vi "Receive Results Object.vi"(8 "error in (no error)":errorcluster, 10 "Results.lvclass":refnum<class "Results.lvclass">, 11 "Controller in":refnum<class "Controller.lvclass">) -> (0 "error out":errorcluster, 3 "Controller out":refnum<class "Controller.lvclass">)   [LabVIEW 2015, in "Controller Actor.lvlib" / "Controller.lvclass"]
uses:
  Controller.lvclass
  Results/Results.lvclass
  Results/Results.lvclass/Results.ctl
  <vilib>/ActorFramework/Message Enqueuer/Message Enqueuer.lvclass/Message Enqueuer.ctl
  <vilib>/ActorFramework/Message Enqueuer/Enqueue.vi
  <vilib>/ActorFramework/Message Priority Queue/Priority Enqueue.vi
  <vilib>/ActorFramework/Stop Msg/Stop Msg.lvclass
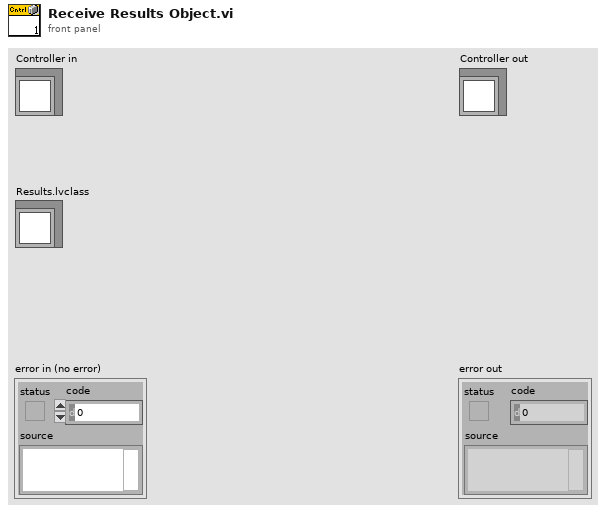
[diagram p1: front panel]
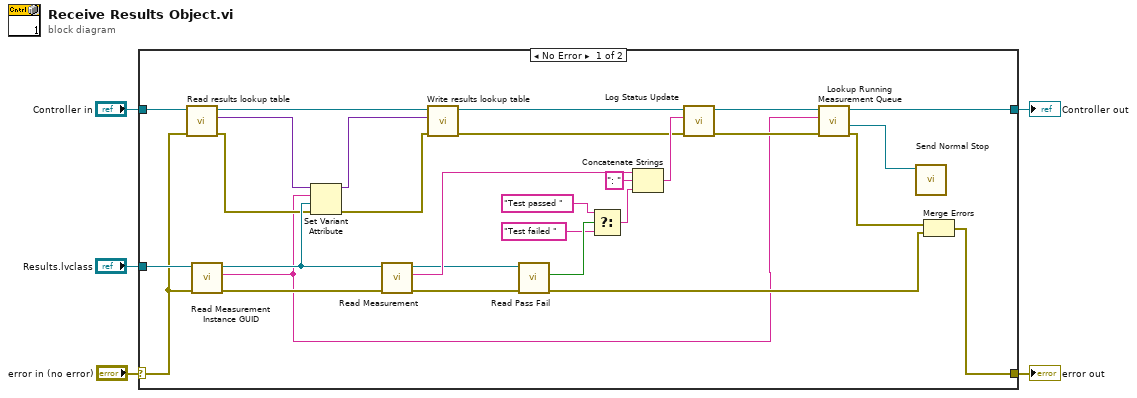
[diagram p0: block diagram]
diagram:
  n1 = case shown="No Error" "error in (no error)" {
    selector: "error in (no error)" -> [w6 w36]
    tunnel: [w9 w36] -> w4
    tunnel: [w19 w35] -> w2
    tunnel: "Controller in" -> [w8 w35]
    tunnel: "Results.lvclass" -> [w21 _]
    frame No Error {
      n2 = call "Read results lookup table.vi"("error in (no error)"=w6, "Controller in"=w8) -> ("error out"=w17:errorcluster, "results lookup table (measurement.timestamp -> results object)"=w34:variant, "Controller out"=w33:refnum<class "Controller.lvclass">)  [unwired: 7 in]
      n3 = call "Read Measurement Instance GUID.vi"("error in (no error)"=w6, "Results in"=w21) -> ("error out"=w13:errorcluster, "Measurement Instance GUID"=w7:string, "Results out"=w31:refnum<class "Results.lvclass">)  [unwired: 7 in]
      n4 = Set Variant Attribute(Variant=w34, name=w7, value=w31, error in=w17) -> (Variant out=w32:variant, error out=w16:errorcluster)  [unwired: 1 out]
      n5 = call "Read Measurement.vi"("error in (no error)"=w13, "Results in"=w31) -> ("error out"=w12:errorcluster, "Measurement"=w28:string, "Results out"=w27:refnum<class "Results.lvclass">)  [unwired: 7 in]
      n6 = call "Write results lookup table.vi"("error in (no error)"=w16, "results lookup table (measurement.timestamp -> results object)"=w32, "Controller in"=w33) -> ("error out"=w15:errorcluster, "Controller out"=w30:refnum<class "Controller.lvclass">)  [unwired: 7 in]
      n7 = call "Read Pass Fail.vi"("error in (no error)"=w12, "Results in"=w27) -> ("error out"=w11:errorcluster, "Pass Fail"=w24:bool)  [unwired: 7 in, 1 out]
      n8 = Select(t="Test passed " ("string"), s=w24, f="Test failed " ("string")) -> (s? t:f=w25:string)
      n9 = Concatenate Strings(w28, ": " ("string"), w25) -> (w29:string)
      n10 = call-dynamic "Log Status Update.vi"("error in (no error)"=w15, "String"=w29, "Controller in"=w30) -> ("error out"=w14:errorcluster, "Controller out"=w20:refnum<class "Controller.lvclass">)  [unwired: 7 in]
      n11 = call "Lookup Running Measurement Queue.vi"("error in (no error)"=w14, "Measurement Name.Harware()"=w7, "Controller in"=w20) -> ("error out"=w10:errorcluster, "Measurement Queue"=w18:refnum<class "Message Enqueuer.lvclass">, "Controller out"=w19:refnum<class "Controller.lvclass">)  [unwired: 5 in, 1 out]
      n12 = call <vilib>:"Send Normal Stop.vi"("Message Enqueuer"=w18) -> ()  [unwired: 10 in, 1 out]
      n13 = Merge Errors(w10, w11) -> (w9:errorcluster)
    }
    frame Error {
    }
  }
  "error out" <- w4
  "Controller out" <- w2
